vi "read_data.vi"(8 "error in (no error)":errorcluster, 11 "SpectralCoclustering in":refnum<class "SpectralCoclustering.lvclass">) -> (0 "error out":errorcluster, 2 "data":T1, 3 "SpectralCoclustering out":refnum<class "SpectralCoclustering.lvclass">)   [LabVIEW 2020, in "SpectralCoclustering.lvclass"]
uses:
  SpectralCoclustering.lvclass
  Controls/spectral_coclustering_data.ctl
  SpectralCoclustering.lvclass/SpectralCoclustering.ctl
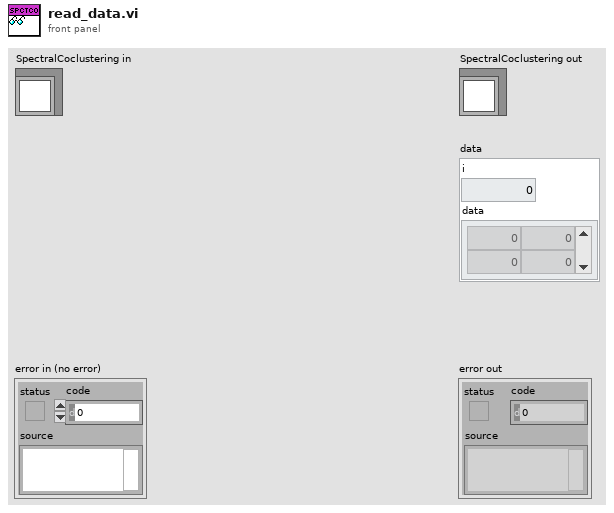
[diagram p1: front panel]
types:
  T1 = typedef "spectral_coclustering_data.ctl" = cluster{"i":dbl, "data":dbl[][]}
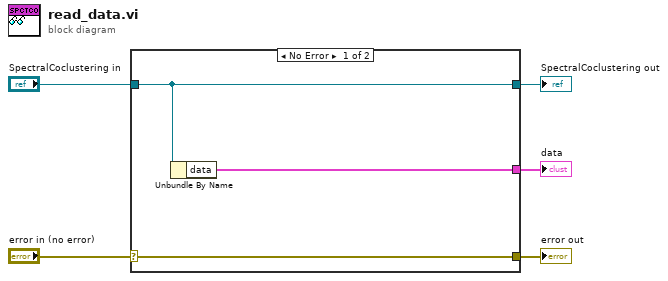
[diagram p0: block diagram]
diagram:
  n1 = case shown="No Error" "error in (no error)" {
    selector: "error in (no error)" -> [w8 w9]
    tunnel: [w8 w9] -> w4
    tunnel: [w7 w10] -> w2
    tunnel: "SpectralCoclustering in" -> [w7 w10]
    tunnel: [w6 _] -> w1
    frame No Error {
      n2 = Unbundle By Name(w7) -> ("data"=w6:T1)
    }
    frame Error {
    }
  }
  "error out" <- w4
  "SpectralCoclustering out" <- w2
  "data" <- w1
